vi "Actor Core.vi"(8 "error in":errorcluster, 11 "DemoAppBar in":refnum<class "DemoAppBar.lvclass">) -> (0 "error out":errorcluster, 3 "Actor out":refnum<class "Actor.lvclass">)   [LabVIEW 2012, in "Win8uiDemo.lvlib" / "DemoAppBar.lvclass"]
doc: "(<B>Filename</B>: Actor Framework.lvlib:Actor.lvclass:Actor Core.vi)\n\nReceives messages to the actor, reacts to them, and initiates any error handling that may shut the actor down.\n\nDescendant classes may override this VI to append parallel tasks for the actor to complete while it handles messages. Overrides use the Call Parent Method node."
uses:
  DemoAppBar.lvclass
  <vilib>/ActorFramework/Actor/Actor.lvclass
  Win8uiFramework/AppBarView.lvclass
  <vilib>/ActorFramework/Actor/Actor.lvclass/Actor.ctl
  <vilib>/ActorFramework/Message Enqueuer/Message Enqueuer.lvclass/Message Enqueuer.ctl
  Win8uiFramework/ViewableActor.lvclass/ViewableActor.ctl
  DemoMain Messages/Start Sensor Msg/Start Sensor Msg.lvclass/Start Sensor Msg.ctl
  Win8uiFramework/Read Stop Event.vi
  <vilib>/ActorFramework/Message Enqueuer/Init from Existing Queue.vi
  <vilib>/ActorFramework/Message Enqueuer/Enqueue.vi
  <vilib>/ActorFramework/Message Priority Queue/Priority Enqueue.vi
  <vilib>/ActorFramework/Message Enqueuer/Message Enqueuer.lvclass
  <vilib>/ActorFramework/Stop Msg/Stop Msg.lvclass
  DemoMain Messages/Start Sensor Msg/Start Sensor Msg.lvclass
  Win8uiFramework/ViewableActor.lvclass
  Flyout/Flyout.lvclass
panel:
  in  "Add":bool
  in  "Quit":bool
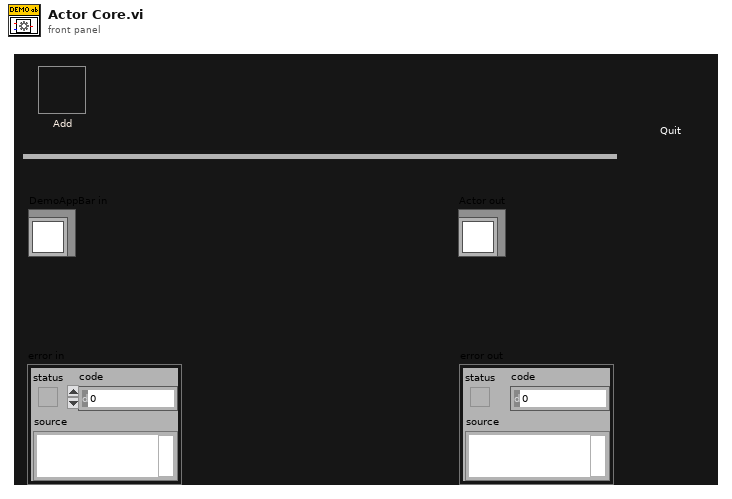
[diagram p1: front panel]
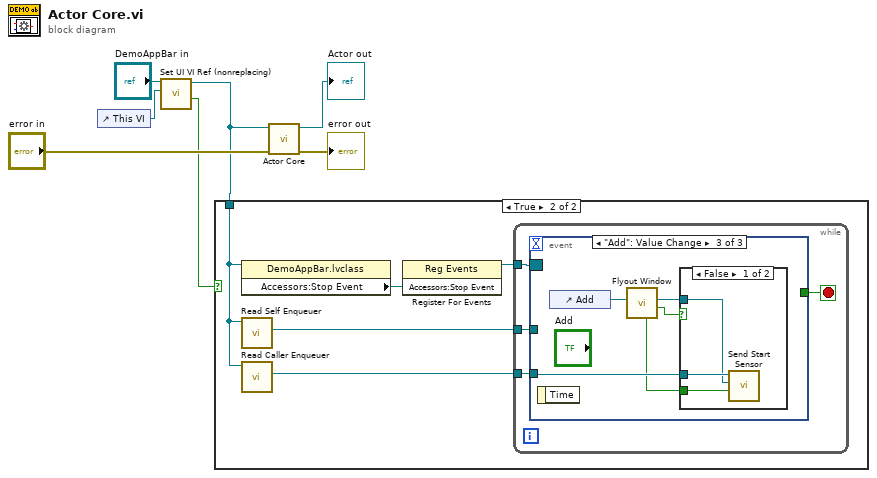
[diagram p0: block diagram]
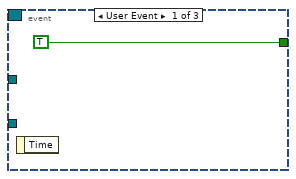
[diagram p3: hidden frame]
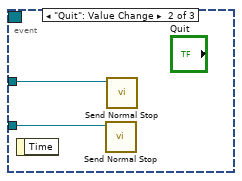
[diagram p4: hidden frame]
diagram:
  n1 = control-ref of="This VI"() -> (w3:refnum<vi>)
  n2 = call "Set UI VI Ref (nonreplacing).vi"("UI VI Ref"=w3, "ViewableActor in"="DemoAppBar in") -> ("Top Level UI?"=w2:bool, "ViewableActor out"=w1:refnum<class "DemoAppBar.lvclass">)  [unwired: 7 in, 1 out]
  n3 = case shown="True" w2 {
    tunnel: w1 -> [_ w10]
    frame False {
    }
    frame True {
      n4 = property class="DemoAppBar.lvclass"(reference=w10) -> ("Accessors:Stop Event"=w12:refnum<user-event>)  [unwired: 1 in, 2 out]
      n5 = call <vilib>:"Read Self Enqueuer.vi"("Actor"=w10) -> ("Self Enqueuer"=w8:refnum<class "Message Enqueuer.lvclass">)  [unwired: 10 in]
      n6 = call <vilib>:"Read Caller Enqueuer.vi"("Actor"=w10) -> ("Caller Enqueuer"=w9:refnum<class "Message Enqueuer.lvclass">)  [unwired: 10 in]
      n7 = register-events(w12) -> (reference out=w11:refnum<event-registration>)  [unwired: 2 in, 1 out]
      n8 = while {
        tunnel: w11 -> [w16]
        tunnel: w9 -> [w14]
        tunnel: w8 -> [w13]
        stop <- w15 stop-if-true
        n9 = event shown="[2] \"Add\": Value Change" {
          selector: w16 -> [_ _ _]
          dyn-events: _ -> [_ _ _]
          timeout: _ -> [_ _ _]
          tunnel: [TRUE _ _] -> w15
          tunnel: w14 -> [_ w19 w24]
          tunnel: w13 -> [_ w18 _]
          event User Event {
            n10 = event-data() -> ()  [unwired: 1 in, 1 out]
          }
          event "Quit": Value Change {
            n11 = event-data() -> ()  [unwired: 1 in, 1 out]
            n12 = call <vilib>:"Send Normal Stop.vi"("Message Enqueuer"=w19) -> ()  [unwired: 10 in, 1 out]
            n13 = call <vilib>:"Send Normal Stop.vi"("Message Enqueuer"=w18) -> ()  [unwired: 10 in, 1 out]
          }
          event "Add": Value Change {
            n14 = event-data() -> ()  [unwired: 1 in, 1 out]
            n15 = control-ref of="Add"() -> (w23:refnum<vi>)
            n16 = call "Flyout Window.vi"("Boolean in"=w23) -> ("Cancelled?"=w22:bool, "Sensor Out"=w21:refnum<class "Sensor.lvclass">, "AutoStart?"=w20:bool)  [unwired: 8 in]
            n17 = case shown="False" w22 {
              tunnel: w24 -> [w27 _]
              tunnel: w21 -> [w26 _]
              tunnel: w20 -> [w25 _]
              frame False {
                n18 = call "Send Start Sensor.vi"("AutoStart? (T)"=w25, "Sensor"=w26, "Message Enqueuer"=w27) -> ()  [unwired: 7 in, 2 out]
              }
              frame True {
              }
            }
          }
        }
      }
    }
  }
  n19 = call-parent "Actor Core.vi"("error in"="error in", "AppBarView in"=w1) -> ("error out"=→"error out":errorcluster, "Actor out"=→"Actor out":refnum<class "Actor.lvclass">)  [unwired: 8 in]
